vi "Direct Control Data Interaction.vi"(5 "mode":enum16{"Init", "read", "write"}(ring), 7 "工位数":u8, 9 "玻璃Hall清零输入":bool[](array[boolean]), 10 "电流值输入":sgl[](array[numeric]), 11 "玻璃当前Hall输入":i64[](array[numeric])) -> (1 "电流值输出":sgl[](array[numeric]), 2 "玻璃Hall清零输出":bool[](array[boolean]), 3 "玻璃当前Hall输出":i64[](array[numeric]))   [LabVIEW 2018]
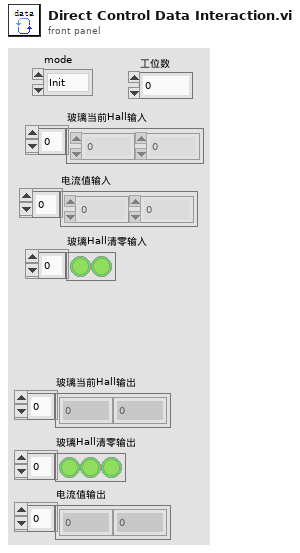
[diagram p1: front panel]
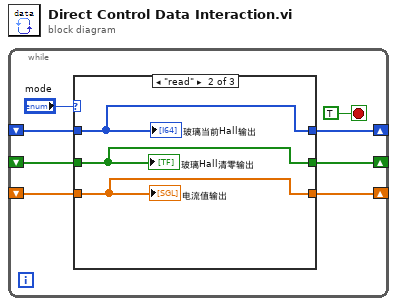
[diagram p0: block diagram]
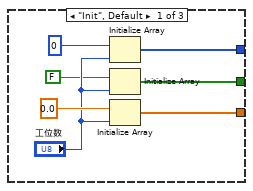
[diagram p2: hidden frame]
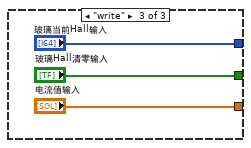
[diagram p3: hidden frame]
diagram:
  n1 = while {
    shift-right: [w7] -> _
    shift-left: _ -> [w5]
    shift-right: [w6] -> _
    shift-left: _ -> [w4]
    shift-right: [w2] -> _
    shift-left: _ -> [w1]
    stop <- TRUE stop-if-true
    n2 = case shown="\"read\"" "mode" {
      tunnel: [w14 w18 "玻璃当前Hall输入"] -> w7
      tunnel: [w13 w17 "玻璃Hall清零输入"] -> w6
      tunnel: w5 -> [_ w18 _]
      tunnel: w4 -> [_ w17 _]
      tunnel: [w11 w16 "电流值输入"] -> w2
      tunnel: w1 -> [_ w16 _]
      frame "Init", Default {
        n3 = Initialize Array(i64 0 ("玻璃当前Hall"), "工位数") -> (w14:i64[])
        n4 = Initialize Array(FALSE ("玻璃Hall清零"), "工位数") -> (w13:bool[])
        n5 = Initialize Array(sgl 0.0, "工位数") -> (w11:sgl[])
      }
      frame "read" {
        "玻璃当前Hall输出" <- w18
        "玻璃Hall清零输出" <- w17
        "电流值输出" <- w16
      }
      frame "write" {
      }
    }
  }
